vi "getPatternList.vi"(8 "error in":errorcluster, 10 "StationId":u32) -> (0 "error out":errorcluster, 3 "TemplatePaths":path[](array[path]))   [LabVIEW 2018]
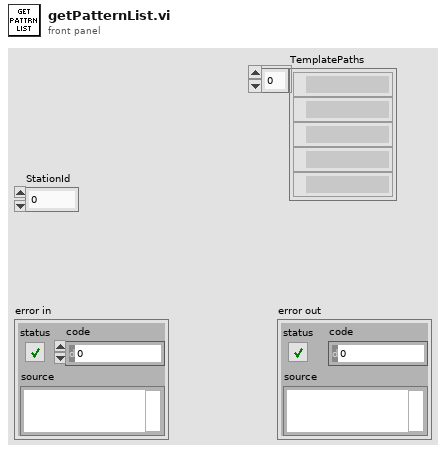
[diagram p1: front panel]
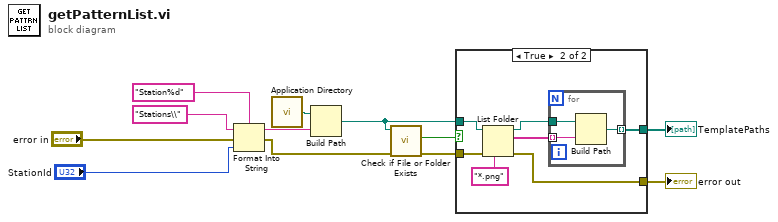
[diagram p0: block diagram]
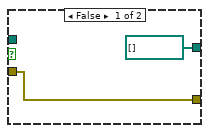
[diagram p2: hidden frame]
diagram:
  n1 = Format Into String(format string="Station%d", initial string="Stations\\" ("name or relative path"), error in="error in", "StationId") -> (resulting string=w8:string, error out=w4:errorcluster)
  n2 = call <vilib>:"Application Directory.vi"() -> ("Application Directory"=w12:path)
  n3 = Build Path(base path=w12, name or relative path=w8) -> (appended path=w2:path)
  n4 = call <vilib>:"Check if File or Folder Exists.vi"("error in (no error)"=w4, "path"=w2) -> ("error out"=w3:errorcluster, "file or folder exists?"=w1:bool)  [unwired: 7 in, 1 out]
  n5 = case shown="True" w1 {
    tunnel: [path[] [] w19] -> w7
    tunnel: [w13 w18] -> w5
    tunnel: w3 -> [w13 w17]
    tunnel: w2 -> [_ w16]
    frame False {
    }
    frame True {
      n6 = List Folder(path=w16, pattern="*.png", error in=w17) -> (path out=w15:path, filenames=w20:string[], error out=w18:errorcluster)  [unwired: 1 in, 1 out]
      n7 = for {
        tunnel: w15 -> [w24]
        tunnel: w20 -> [w23] mode=indexing
        tunnel: [w22] -> w19 mode=indexing
        n8 = Build Path(base path=w24, name or relative path=w23) -> (appended path=w22:path)
      }
    }
  }
  "TemplatePaths" <- w7
  "error out" <- w5
